vi "Get Accel Value.vi"(11 "drive.lvclass":refnum<class "drive.lvclass">) -> (2 "Y-Axis":dbl, 3 "drive.lvclass":refnum<class "drive.lvclass">)   [LabVIEW 2015, in "drive.lvclass"]
uses:
  drive.lvclass
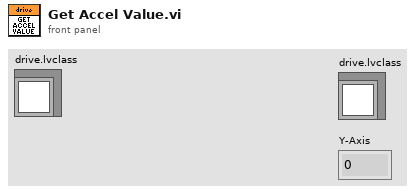
[diagram p1: front panel]
types:
  T1 = typedef "WPI_AccelerometerDevRef.ctl" = cluster{"DevStatus":errorcluster, "Scaling":T2, "Analog Channels":T3, "I2C Bus":T5, "SPI Bus":T6, "Accel Range":T7, "ADXL Axes":T8, "Handle":i32, "Device Address":u8, "Accel Type":enum16{"Analog", "ADXL345 I2C", "ADXL345 SPI", "Internal", "ADXL362 SPI"}}
  T2 = typedef "WPI_AccelerometerScaling.ctl" = cluster{"Gain (VoltsPerG)":dbl, "Center Voltage":dbl}
  T3 = typedef "WPI_AccelerometerAnalogChannels.ctl" = cluster{"X-Axis":T4, "Y-Axis":T4, "Z-Axis":T4}
  T4 = typedef "FPGA_AIChannel.ctl" = enum8{"AI 0", "AI 1", "AI 2", "AI 3", "AI MXP 0", "AI MXP 1", "AI MXP 2", "AI MXP 3", "Invalid"}
  T5 = typedef "i2c_bus.ctl" = enum16{"I2C On-Board", "I2C MXP", "Invalid"}
  T6 = typedef "spi_bus.ctl" = enum16{"SPI On-Board, CS0", "SPI On-Board, CS1", "SPI On-Board, CS2", "SPI On-Board, CS3", "SPI MXP", "Invalid"}
  T7 = typedef "ADXL345 Range.ctl" = u8
  T8 = typedef "WPI_AccelerometerADXL345 Axes.ctl" = cluster{"X-Axis":bool, "Y-Axis":bool, "Z-Axis":bool}
  T9 = cluster{"X-Axis":dbl, "Y-Axis":dbl, "Z-Axis":dbl}
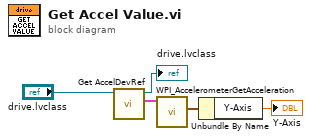
[diagram p0: block diagram]
diagram:
  n1 = call-dynamic "Get AccelDevRef.vi"("drive in"="drive.lvclass") -> ("AccelerometerDevRef"=w4:T1, "drive out"=→"drive.lvclass":refnum<class "drive.lvclass">)  [unwired: 8 in, 1 out]
  n2 = call <vilib>:"WPI_AccelerometerGetAcceleration.vi"("AccelerometerDevRef"=w4) -> ("Accelerations"=w3:T9)  [unwired: 8 in, 2 out]
  n3 = Unbundle By Name(w3) -> ("Y-Axis"=→"Y-Axis":dbl)
